vi "SubVI - Receive Config File.vi"(11 "file path (use dialog)":path) -> (0 "error out":errorcluster)   [LabVIEW 2017]
panel:
  out "Progress ( % )":u8
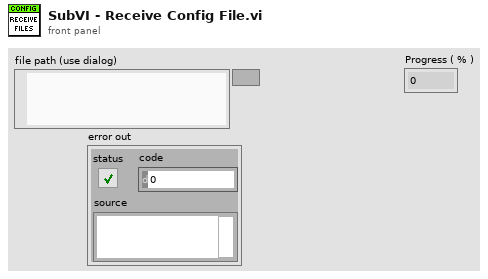
[diagram p1: front panel]
types:
  T1 = enum16{"open", "replace", "create", "open or create", "replace or create", "replace or create with confirmation"}
  T2 = enum16{"big-endian, network order", "native, host order", "little-endian"}
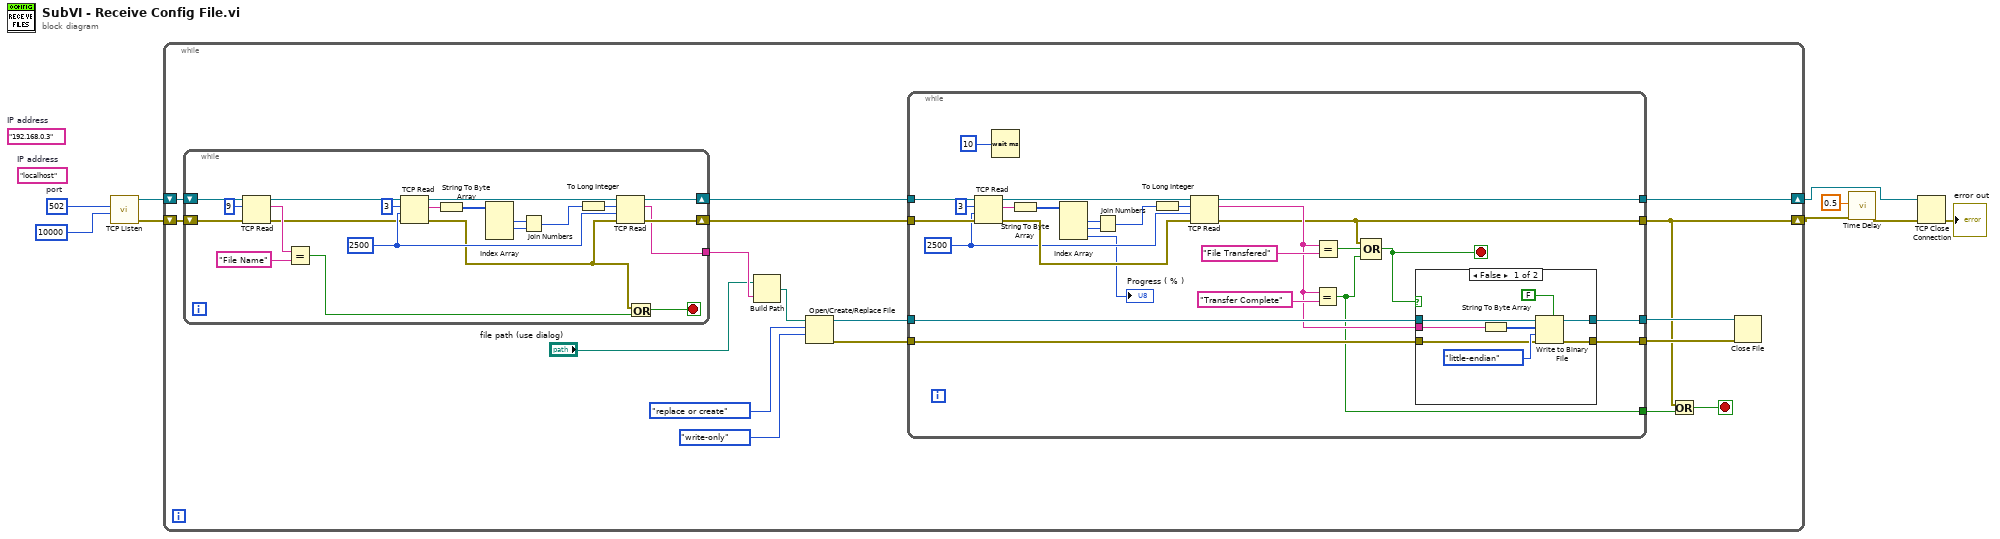
[diagram p0: block diagram]
diagram:
  (unwired) "192.168.0.3"  # IP address
  w9 = u16 502  # port
  (unwired) "localhost"  # IP address
  n1 = call <vilib>:"TCP Listen.vi"("timeout ms (wait forever: -1)"=10000, "port"=w9) -> ("error out"=w6:errorcluster, "connection ID"=w7:refnum<k5>)  [unwired: 5 in, 3 out]
  n2 = while {
    shift-right: [w13] -> w5
    shift-left: w7 -> [w20]
    shift-right: [w10] -> w4
    shift-left: w6 -> [w22]
    stop <- w11 stop-if-true
    n3 = while {
      shift-right: [w31] -> w21
      shift-left: w22 -> [w45]
      shift-right: [w32] -> w19
      shift-left: w20 -> [w44]
      tunnel: [w29] -> w18
      stop <- w28 stop-if-true
      w35 = 2500 ("timeout ms (25000)")
      n4 = TCP Read(connection ID=w44, bytes to read=9, error in (no error)=w45) -> (connection ID out=w34:refnum<k5>, data out=w47:string, error out=w33:errorcluster)  [unwired: 2 in]
      n5 = Equal?(x=w47, y="File Name" ("data in")) -> (x = y?=w30:bool)
      n6 = TCP Read(connection ID=w34, bytes to read=3, error in (no error)=w33, 9:w35) -> (connection ID out=w38:refnum<k5>, data out=w42:string, error out=w27:errorcluster)  [unwired: 1 in]
      n7 = String To Byte Array(string=w42) -> (unsigned byte array=w41:u8[])
      n8 = Index Array(array=w41) -> (element #1=w40:u8, element #2=w39:u8)  [unwired: 3 in, 1 out]
      n9 = Join Numbers(hi=w40, lo=w39) -> ((hi.lo)=w36:u16)
      n10 = To Long Integer(number=w36) -> (32bit integer=w37:i32)
      n11 = TCP Read(connection ID=w38, bytes to read=w37, error in (no error)=w27, 9:w35) -> (connection ID out=w32:refnum<k5>, data out=w29:string, error out=w31:errorcluster)  [unwired: 1 in]
      n12 = Or(x=w27, y=w30) -> (x .or. y?=w28:bool)
    }
    n13 = Build Path(base path="file path (use dialog)", name or relative path=w18) -> (appended path=w16:path)
    n14 = Open/Create/Replace File(file path (use dialog)=w16, operation (0:open)=T1."replace or create", access (0:read/write)=enum16{"read/write", "read-only", "write-only"}."write-only") -> (refnum out=w23:refnum<file>, error out=w24:errorcluster)  [unwired: 3 in, 1 out]
    n15 = while {
      tunnel: w19 -> [w74]
      tunnel: w21 -> [w73]
      tunnel: [w64] -> w13
      tunnel: [w49] -> w10
      tunnel: w24 -> [w62]
      tunnel: w23 -> [w61]
      tunnel: [w60] -> w14
      tunnel: [w59] -> w15
      tunnel: [w50] -> w12
      stop <- w51 stop-if-true
      w56 = 2500 ("timeout ms (25000)")
      n16 = TCP Read(connection ID=w74, bytes to read=3, error in (no error)=w73, 9:w56) -> (connection ID out=w67:refnum<k5>, data out=w71:string, error out=w66:errorcluster)  [unwired: 1 in]
      n17 = Wait (ms)(milliseconds to wait=u32 10) -> ()  [unwired: 1 out]
      n18 = String To Byte Array(string=w71) -> (unsigned byte array=w70:u8[])
      n19 = Index Array(array=w70) -> (element #1=w69:u8, element #2=w68:u8, element #3=→"Progress ( % )":u8)  [unwired: 3 in]
      n20 = Join Numbers(hi=w69, lo=w68) -> ((hi.lo)=w57:u16)
      n21 = To Long Integer(number=w57) -> (32bit integer=w65:i32)
      n22 = TCP Read(connection ID=w67, bytes to read=w65, error in (no error)=w66, 9:w56) -> (connection ID out=w64:refnum<k5>, data out=w52:string, error out=w49:errorcluster)  [unwired: 1 in]
      n23 = Equal?(x=w52, y="Transfer Complete" ("data in")) -> (x = y?=w50:bool)
      n24 = Equal?(x=w52, y="File Transfered" ("data in")) -> (x = y?=w58:bool)
      n25 = Compound Arithmetic op=OR(w49, w58, w50) -> (w51:bool)
      n26 = case shown="False" w51 {
        tunnel: w62 -> [w80 w83]
        tunnel: w61 -> [w79 w84]
        tunnel: [w78 w84] -> w60
        tunnel: [w77 w83] -> w59
        tunnel: w52 -> [w76 _]
        frame False {
          n27 = String To Byte Array(string=w76) -> (unsigned byte array=w75:u8[])
          n28 = Write to Binary File(file (use dialog)=w79, data=w75, error in=w80, 5:FALSE ("prepend array or string size? (T)"), 9:T2."little-endian" ("byte order (0:big-endian, network order)")) -> (refnum out=w78:refnum<file>, error out=w77:errorcluster)  [unwired: 1 in, 1 out]
        }
        frame True {
        }
      }
    }
    n29 = Or(x=w10, y=w12) -> (x .or. y?=w11:bool)
    n30 = Close File(refnum=w14, error in=w15) -> ()  [unwired: 2 out]
  }
  n31 = call "Time Delay"("error in (no error)"=w4, "Delay Time (s)"=0.5) -> ("error out"=w3:errorcluster)  [unwired: 9 in]
  n32 = TCP Close Connection(connection ID=w5, error in (no error)=w3) -> (error out=→"error out":errorcluster)  [unwired: 1 in, 1 out]
